vi "Rename Constants.vi"(8 "error in (no error)":errorcluster, 10 "VI Reference in":refnum<vi>, 11 "ProjectItem in":refnum<class "ProjectItem.lvclass">) -> (0 "error out":errorcluster, 1 "Changed?":bool, 2 "VI Reference out":refnum<vi>, 3 "ProjectItem out":refnum<class "ProjectItem.lvclass">)   [LabVIEW 2019, in "ProjectItem.lvclass"]
uses:
  ProjectItem.lvclass
  <vilib>/Utility/traverseref.llb/TRef TravTarget.ctl
  <vilib>/Utility/traverseref.llb/VI Scripting - Traverse.lvlib
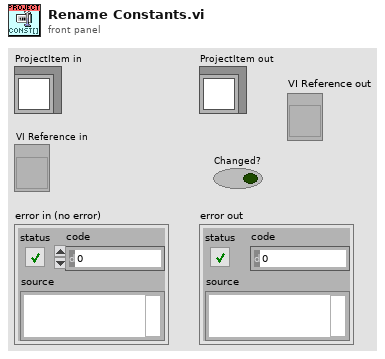
[diagram p1: front panel]
types:
  T1 = typedef "TRef TravTarget.ctl" = enum16{"FP", "BD", "Other"}
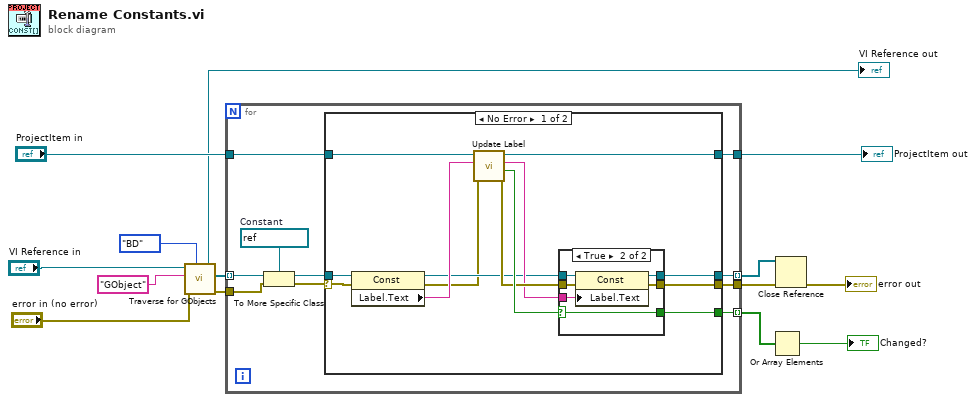
[diagram p0: block diagram]
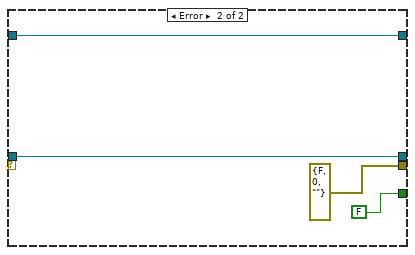
[diagram p3: hidden frame]
diagram:
  n1 = call <vilib>:"Traverse for GObjects.vi"("Traverse Target"=TRef_TravTarget."BD", "error in (no error)"="error in (no error)", "Class Name"="GObject", "VI Refnum"="VI Reference in") -> ("error out"=w11:errorcluster, "References"=w7:refnum<vi>[], "dup VI Refnum"=→"VI Reference out":refnum<vi>)  [unwired: 4 in, 1 out]
  n2 = for {
    tunnel: w7 -> [w24] mode=indexing
    tunnel: [w20] -> w8 mode=indexing
    tunnel: "ProjectItem in" -> [w19]
    tunnel: w11 -> [w18]
    tunnel: [w17] -> w12
    tunnel: [w16] -> w13 mode=indexing
    tunnel: [w15] -> w14
    w23 = refnum<vi> refnum  # Constant
    n3 = To More Specific Class(target class=w23, reference=w24, error in=w18) -> (specific class reference=w21:refnum<vi>, error out=w22:errorcluster)
    n4 = case shown="No Error" w22 {
      selector: w22 -> [w29 _]
      tunnel: w21 -> [w37 w50]
      tunnel: [w27 w50] -> w20
      tunnel: w19 -> [w33 w49]
      tunnel: [w28 w49] -> w17
      tunnel: [w26 FALSE] -> w16
      tunnel: [w25 errorcluster {"status"=FALSE, "code"=0, "source"=""} ("error out")] -> w15
      frame No Error {
        n5 = property class="Const"(reference=w37, error in=w29) -> (reference out=w31:refnum<vi>, error out=w30:errorcluster, "Label.Text"=w32:string)
        n6 = call "Update Label.vi"("error in (no error)"=w30, "Label in"=w32, "Rename in"=w33) -> ("error out"=w35:errorcluster, "New Label?"=w36:bool, "Label out"=w34:string, "Rename out"=w28:refnum<class "ProjectItem.lvclass">)  [unwired: 5 in]
        n7 = case shown="True" w36 {
          selector: w36 -> [w40 w43]
          tunnel: w31 -> [w39 w46]
          tunnel: w34 -> [_ w45]
          tunnel: w35 -> [w38 w44]
          tunnel: [w40 w43] -> w26
          tunnel: [w39 w42] -> w27
          tunnel: [w38 w41] -> w25
          frame False {
          }
          frame True {
            n8 = property class="Const"(reference=w46, error in=w44, "Label.Text"=w45) -> (reference out=w42:refnum<vi>, error out=w41:errorcluster)
          }
        }
      }
      frame Error {
      }
    }
  }
  "ProjectItem out" <- w12
  n9 = Or Array Elements(Boolean array=w13) -> (logical OR=→"Changed?":bool)
  n10 = Close Reference(reference=w8, error in (no error)=w14) -> (error out=→"error out":errorcluster)
